vi "GOOP_GetOverlayIconPath.vi"(11 "IconName(NoPngExtension)":string) -> (3 "IconPath":path)   [LabVIEW 2020]
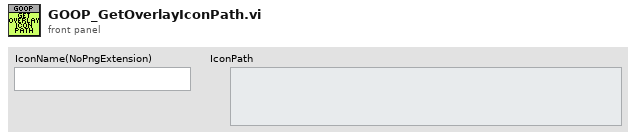
[diagram p1: front panel]
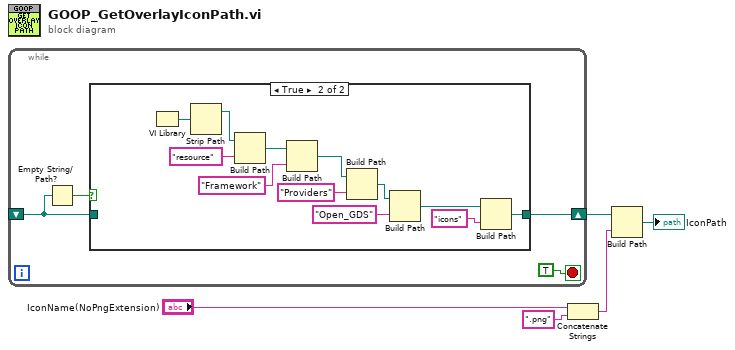
[diagram p0: block diagram]
diagram:
  n1 = while {
    shift-right: [w8] -> w3
    shift-left: _ -> [w7]
    stop <- TRUE stop-if-true
    n2 = Empty String/Path?(string/path=w7) -> (empty?=w9:bool)
    n3 = case shown="True" w9 {
      tunnel: [w10 w12] -> w8
      tunnel: w7 -> [w10 _]
      frame False {
      }
      frame True {
        n4 = VI Library() -> (path=w14:path)
        n5 = Strip Path(path=w14) -> (stripped path=w15:path)  [unwired: 1 out]
        n6 = Build Path(base path=w15, name or relative path="resource") -> (appended path=w16:path)
        n7 = Build Path(base path=w16, name or relative path="Framework") -> (appended path=w17:path)
        n8 = Build Path(base path=w17, name or relative path="Providers") -> (appended path=w22:path)
        n9 = Build Path(base path=w22, name or relative path="Open_GDS") -> (appended path=w11:path)
        n10 = Build Path(base path=w11, name or relative path="icons") -> (appended path=w12:path)
      }
    }
  }
  n11 = Concatenate Strings("IconName(NoPngExtension)", ".png" ("string")) -> (w4:string)
  n12 = Build Path(base path=w3, name or relative path=w4) -> (appended path=→"IconPath":path)
